vi "To Waveform.vi"(8 "error in (no error)":errorcluster, 11 "Waveform Array in":refnum<class "Waveform Array.lvclass">) -> (0 "error out":errorcluster, 1 "Success?":bool, 3 "Waveform Array":waveform(dbl)[](array[waveform]))   [LabVIEW 2020, in "Data.lvlib" / "Waveform Array.lvclass"]
doc: "Interpret 'Data' as a Waveform Array. If impossible 'Success?' is set to FALSE"
uses:
  Waveform Array.lvclass
  Waveform Array.lvclass/Waveform Array.ctl
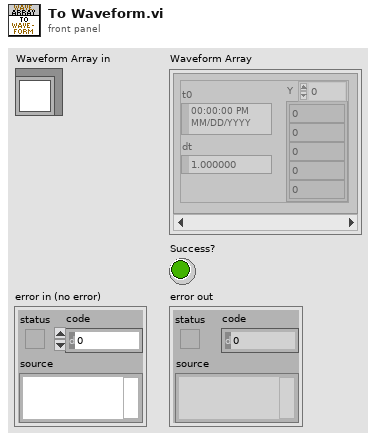
[diagram p1: front panel]
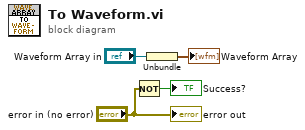
[diagram p0: block diagram]
diagram:
  n1 = Not(x="error in (no error)") -> (.not. x?=→"Success?":bool)
  n2 = Unbundle("Waveform Array in") -> (→"Waveform Array":waveform(dbl)[])
  "error out" <- "error in (no error)"
